vi "TABCheck.vi"(8 "Size":cluster{"X":dbl, "Y":dbl}, 9 "PtIn(Ideal/A)":cluster{"X":dbl, "Y":dbl}, 10 "Robot(B)":cluster{dbl, dbl}[][](array[cluster]), 11 "Ideal(A)":cluster{sgl, sgl}[][](array[cluster])) -> (3 "PtOut(Robot/B)":cluster{"OX":dbl, "OY":dbl})   [LabVIEW 2014]
panel:
  out "PointArray":cluster{"X":i32, "Y":i32}
  out "Array 2":cluster{i32, i32}[](array[cluster])
  out "Cluster":cluster{i32, i32}
  # "80,150"
  # "270,110"
  # "0,0"
  # "X,Y"
  # "107.5,160.8"
  # "0,1"
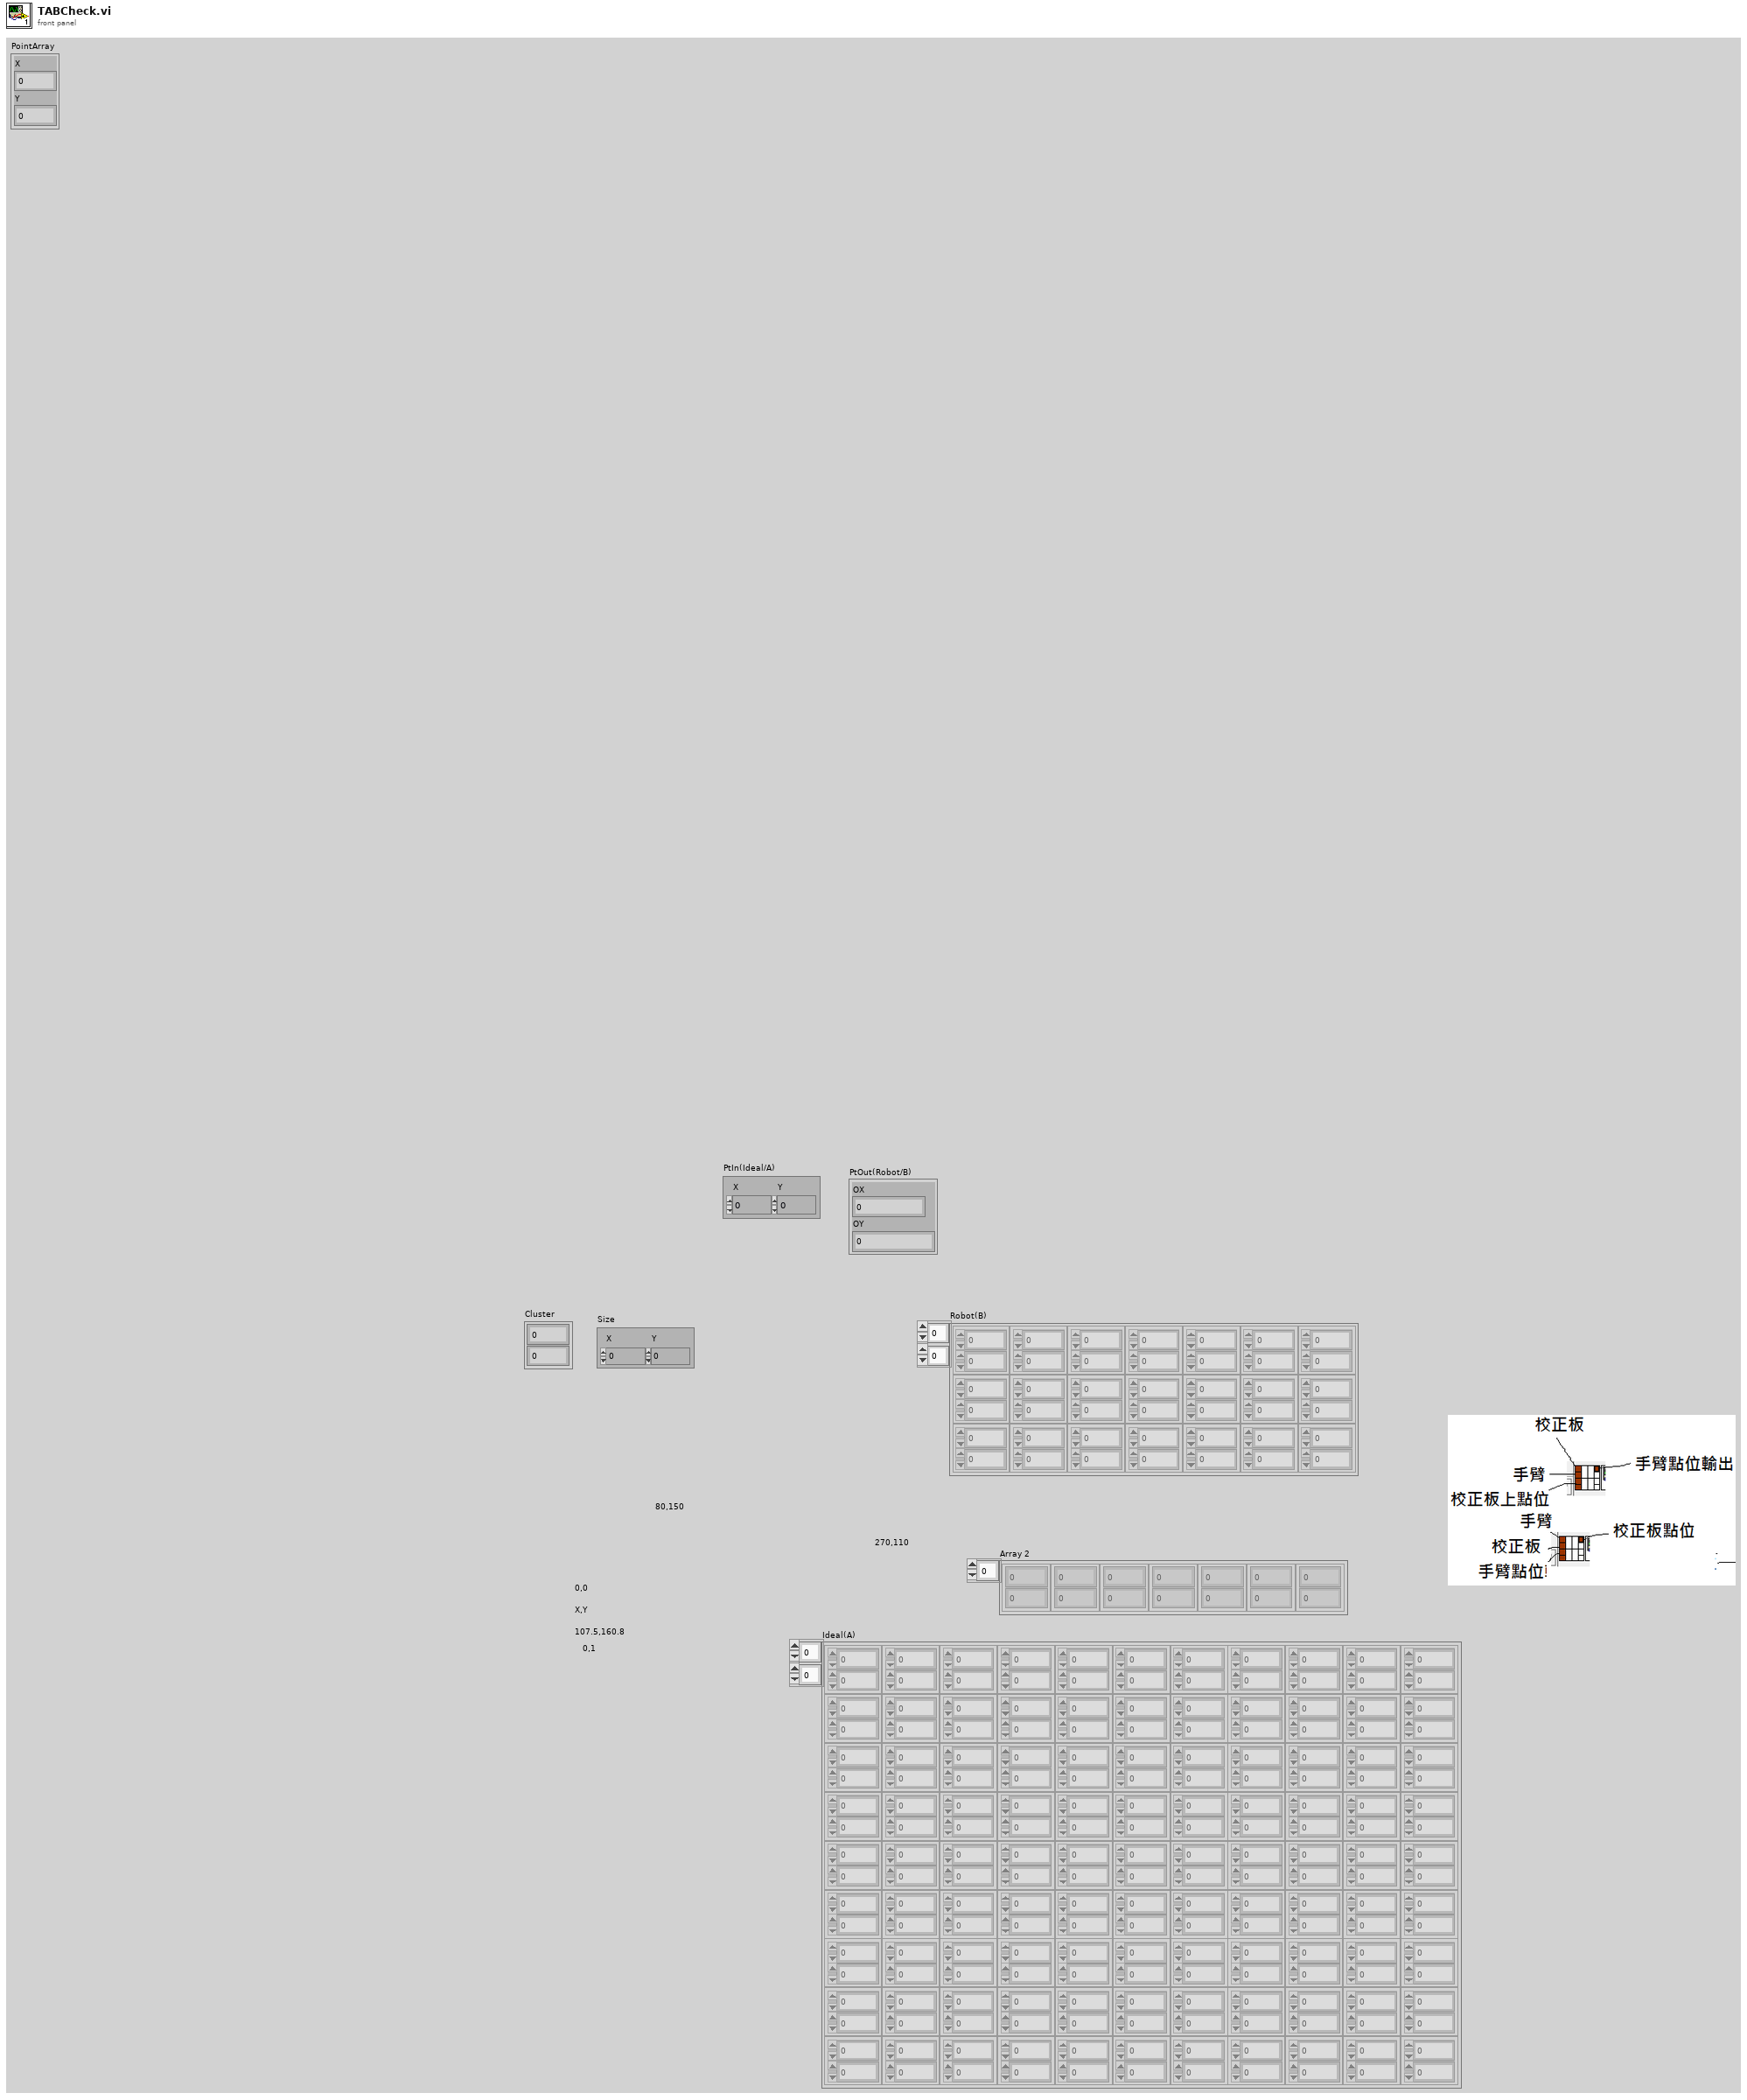
[diagram p1: front panel]
types:
  T1 = cluster{"[0]":sgl, "[1]":sgl, "[2]":sgl, "[3]":sgl}[]
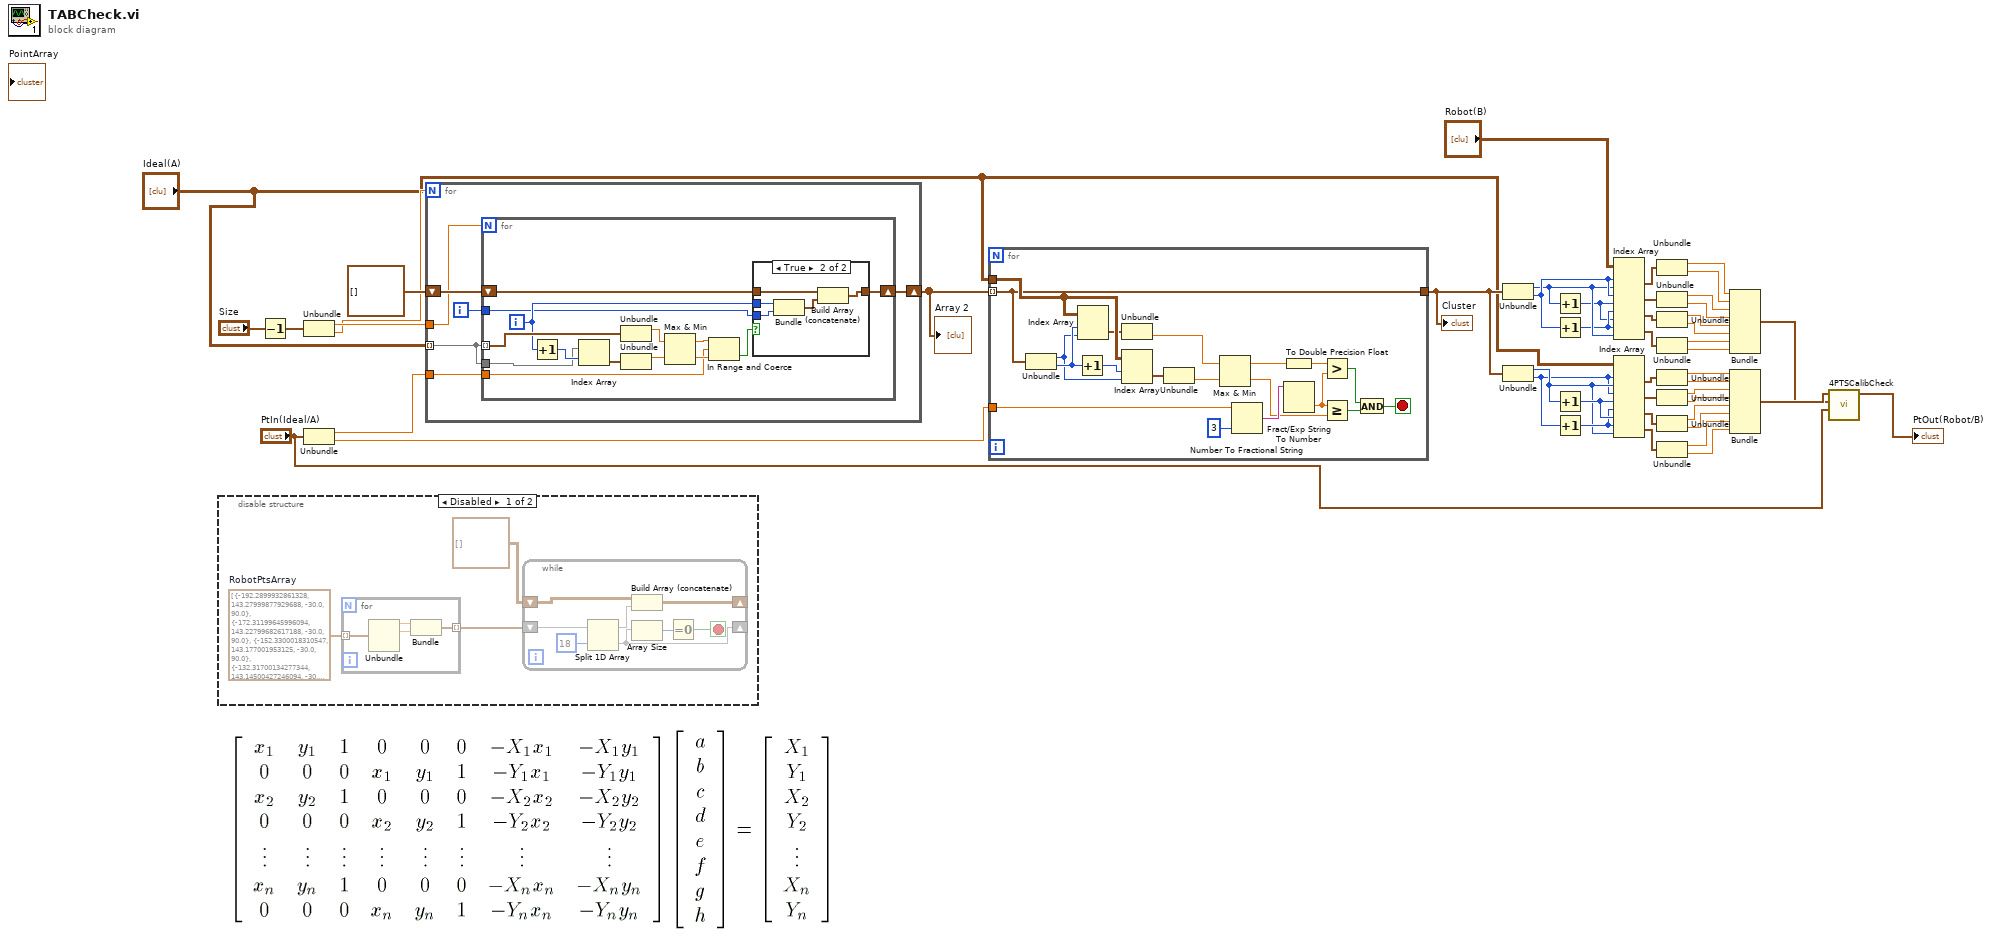
[diagram p0: block diagram]
diagram:
  n1 = disable-structure shown="Disabled" {
    frame Disabled {
      w49 = T1 [{"[0]"=-192.29, "[1]"=143.28, "[2]"=-30.0, "[3]"=90.0}, {"[0]"=-172.312, "[1]"=143.228, "[2]"=-30.0, "[3]"=90.0}, {"[0]"=-152.33, "[1]"=143.177, "[2]"=-30.0, "[3]"=90.0}, {"[0]"=-132.317, "[1]"=143.145, "[2]"=-30.0, "[3]"=90.0}, {"[0]"=-112.255, "[1]"=143.098, "[2]"=-30.0, "[3]"=90.0}, {"[0]"=-92.217, "[1]"=143.035, "[2]"=-30.0, "[3]"=90.0}, {"[0]"=-72.14, "[1]"=142.978, "[2]"=-30.0, "[3]"=90.0}, {"[0]"=-52.078, "[1]"=142.898, "[2]"=-30.0, "[3]"=90.0}, {"[0]"=-31.971, "[1]"=142.795, "[2]"=-30.0, "[3]"=90.0}, {"[0]"=-11.878, "[1]"=142.692, "[2]"=-30.0, "[3]"=90.0}, {"[0]"=8.277, "[1]"=142.568, "[2]"=-30.0, "[3]"=90.0}, {"[0]"=28.398, "[1]"=142.416, "[2]"=-30.0, "[3]"=90.0}, {"[0]"=48.523, "[1]"=142.253, "[2]"=-30.0, "[3]"=90.0}, {"[0]"=68.659, "[1]"=142.079, "[2]"=-30.0, "[3]"=90.0}, {"[0]"=88.714, "[1]"=141.902, "[2]"=-30.0, "[3]"=90.0}, {"[0]"=108.801, "[1]"=141.736, "[2]"=-30.0, "[3]"=90.0}, {"[0]"=128.813, "[1]"=141.58, "[2]"=-30.0, "[3]"=90.0}, {"[0]"=148.873, "[1]"=141.455, "[2]"=-30.0, "[3]"=90.0}, {"[0]"=-192.292, "[1]"=163.166, "[2]"=-30.0, "[3]"=90.0}, {"[0]"=-172.251, "[1]"=163.142, "[2]"=-30.0, "[3]"=90.0}, {"[0]"=-152.315, "[1]"=163.083, "[2]"=-30.0, "[3]"=90.0}, {"[0]"=-132.271, "[1]"=163.04, "[2]"=-30.0, "[3]"=90.0}, {"[0]"=-112.2, "[1]"=162.982, "[2]"=-30.0, "[3]"=90.0}, {"[0]"=-92.147, "[1]"=162.933, "[2]"=-30.0, "[3]"=90.0}, {"[0]"=-72.085, "[1]"=162.842, "[2]"=-30.0, "[3]"=90.0}, {"[0]"=-52.039, "[1]"=162.771, "[2]"=-30.0, "[3]"=90.0}, {"[0]"=-31.931, "[1]"=162.689, "[2]"=-30.0, "[3]"=90.0}, {"[0]"=-11.829, "[1]"=162.589, "[2]"=-30.0, "[3]"=90.0}, {"[0]"=8.306, "[1]"=162.465, "[2]"=-30.0, "[3]"=90.0}, {"[0]"=28.403, "[1]"=162.316, "[2]"=-30.0, "[3]"=90.0}, {"[0]"=48.518, "[1]"=162.165, "[2]"=-30.0, "[3]"=90.0}, {"[0]"=68.639, "[1]"=162.001, "[2]"=-30.0, "[3]"=90.0}, {"[0]"=88.711, "[1]"=161.847, "[2]"=-30.0, "[3]"=90.0}, {"[0]"=108.808, "[1]"=161.693, "[2]"=-30.0, "[3]"=90.0}, {"[0]"=128.797, "[1]"=161.532, "[2]"=-30.0, "[3]"=90.0}, {"[0]"=148.812, "[1]"=161.411, "[2]"=-30.0, "[3]"=90.0}, {"[0]"=-192.201, "[1]"=183.166, "[2]"=-30.0, "[3]"=90.0}, {"[0]"=-172.2, "[1]"=183.08, "[2]"=-30.0, "[3]"=90.0}, {"[0]"=-152.214, "[1]"=183.041, "[2]"=-30.0, "[3]"=90.0}, {"[0]"=-132.197, "[1]"=182.996, "[2]"=-30.0, "[3]"=90.0}, {"[0]"=-112.1, "[1]"=182.941, "[2]"=-30.0, "[3]"=90.0}, {"[0]"=-92.071, "[1]"=182.879, "[2]"=-30.0, "[3]"=90.0}, {"[0]"=-71.982, "[1]"=182.794, "[2]"=-30.0, "[3]"=90.0}, {"[0]"=-51.944, "[1]"=182.709, "[2]"=-30.0, "[3]"=90.0}, {"[0]"=-31.857, "[1]"=182.624, "[2]"=-30.0, "[3]"=90.0}, {"[0]"=-11.772, "[1]"=182.522, "[2]"=-30.0, "[3]"=90.0}, {"[0]"=8.361, "[1]"=182.426, "[2]"=-30.0, "[3]"=90.0}, {"[0]"=28.464, "[1]"=182.29, "[2]"=-30.0, "[3]"=90.0}, {"[0]"=48.542, "[1]"=182.127, "[2]"=-30.0, "[3]"=90.0}, {"[0]"=68.669, "[1]"=181.977, "[2]"=-30.0, "[3]"=90.0}, {"[0]"=88.728, "[1]"=181.825, "[2]"=-30.0, "[3]"=90.0}, {"[0]"=108.824, "[1]"=181.664, "[2]"=-30.0, "[3]"=90.0}, {"[0]"=128.779, "[1]"=181.533, "[2]"=-30.0, "[3]"=90.0}, {"[0]"=148.817, "[1]"=181.423, "[2]"=-30.0, "[3]"=90.0}, {"[0]"=-192.153, "[1]"=203.103, "[2]"=-30.0, "[3]"=90.0}, {"[0]"=-172.128, "[1]"=203.051, "[2]"=-30.0, "[3]"=90.0}, {"[0]"=-152.128, "[1]"=203.019, "[2]"=-30.0, "[3]"=90.0}, {"[0]"=-132.124, "[1]"=202.923, "[2]"=-30.0, "[3]"=90.0}, {"[0]"=-112.011, "[1]"=202.898, "[2]"=-30.0, "[3]"=90.0}, {"[0]"=-91.994, "[1]"=202.829, "[2]"=-30.0, "[3]"=90.0}, {"[0]"=-71.908, "[1]"=202.761, "[2]"=-30.0, "[3]"=90.0}, {"[0]"=-51.86, "[1]"=202.669, "[2]"=-30.0, "[3]"=90.0}, {"[0]"=-31.785, "[1]"=202.589, "[2]"=-30.0, "[3]"=90.0}, {"[0]"=-11.679, "[1]"=202.488, "[2]"=-30.0, "[3]"=90.0}, {"[0]"=8.407, "[1]"=202.38, "[2]"=-30.0, "[3]"=90.0}, {"[0]"=28.501, "[1]"=202.252, "[2]"=-30.0, "[3]"=90.0}, {"[0]"=48.585, "[1]"=202.111, "[2]"=-30.0, "[3]"=90.0}, {"[0]"=68.695, "[1]"=201.96, "[2]"=-30.0, "[3]"=90.0}, {"[0]"=88.739, "[1]"=201.807, "[2]"=-30.0, "[3]"=90.0}, {"[0]"=108.837, "[1]"=201.678, "[2]"=-30.0, "[3]"=90.0}, {"[0]"=128.774, "[1]"=201.553, "[2]"=-30.0, "[3]"=90.0}, {"[0]"=148.765, "[1]"=201.458, "[2]"=-30.0, "[3]"=90.0}, {"[0]"=-192.092, "[1]"=223.039, "[2]"=-30.0, "[3]"=90.0}, {"[0]"=-172.061, "[1]"=223.008, "[2]"=-30.0, "[3]"=90.0}, {"[0]"=-152.068, "[1]"=222.956, "[2]"=-30.0, "[3]"=90.0}, {"[0]"=-132.053, "[1]"=222.884, "[2]"=-30.0, "[3]"=90.0}, {"[0]"=-111.943, "[1]"=222.844, "[2]"=-30.0, "[3]"=90.0}, {"[0]"=-91.934, "[1]"=222.779, "[2]"=-30.0, "[3]"=90.0}, {"[0]"=-71.838, "[1]"=222.729, "[2]"=-30.0, "[3]"=90.0}, {"[0]"=-51.82, "[1]"=222.635, "[2]"=-30.0, "[3]"=90.0}, {"[0]"=-31.71, "[1]"=222.553, "[2]"=-30.0, "[3]"=90.0}, {"[0]"=-11.651, "[1]"=222.445, "[2]"=-30.0, "[3]"=90.0}, {"[0]"=8.465, "[1]"=222.341, "[2]"=-30.0, "[3]"=90.0}, {"[0]"=28.524, "[1]"=222.238, "[2]"=-30.0, "[3]"=90.0}, {"[0]"=48.613, "[1]"=222.096, "[2]"=-30.0, "[3]"=90.0}, {"[0]"=68.708, "[1]"=221.951, "[2]"=-30.0, "[3]"=90.0}, {"[0]"=88.759, "[1]"=221.807, "[2]"=-30.0, "[3]"=90.0}, {"[0]"=108.864, "[1]"=221.681, "[2]"=-30.0, "[3]"=90.0}, {"[0]"=128.728, "[1]"=221.571, "[2]"=-30.0, "[3]"=90.0}, {"[0]"=148.809, "[1]"=221.45, "[2]"=-30.0, "[3]"=90.0}, {"[0]"=-192.03, "[1]"=243.008, "[2]"=-30.0, "[3]"=90.0}, {"[0]"=-171.988, "[1]"=242.954, "[2]"=-30.0, "[3]"=90.0}, {"[0]"=-151.979, "[1]"=242.887, "[2]"=-30.0, "[3]"=90.0}, {"[0]"=-131.972, "[1]"=242.819, "[2]"=-30.0, "[3]"=90.0}, {"[0]"=-111.852, "[1]"=242.82, "[2]"=-30.0, "[3]"=90.0}, {"[0]"=-91.857, "[1]"=242.72, "[2]"=-30.0, "[3]"=90.0}, {"[0]"=-71.764, "[1]"=242.658, "[2]"=-30.0, "[3]"=90.0}, {"[0]"=-51.72, "[1]"=242.586, "[2]"=-30.0, "[3]"=90.0}, {"[0]"=-31.666, "[1]"=242.488, "[2]"=-30.0, "[3]"=90.0}, {"[0]"=-11.566, "[1]"=242.391, "[2]"=-30.0, "[3]"=90.0}, {"[0]"=8.484, "[1]"=242.29, "[2]"=-30.0, "[3]"=90.0}, {"[0]"=28.563, "[1]"=242.187, "[2]"=-30.0, "[3]"=90.0}, {"[0]"=48.663, "[1]"=242.057, "[2]"=-30.0, "[3]"=90.0}, {"[0]"=68.733, "[1]"=241.919, "[2]"=-30.0, "[3]"=90.0}, {"[0]"=88.775, "[1]"=241.787, "[2]"=-30.0, "[3]"=90.0}, {"[0]"=108.887, "[1]"=241.655, "[2]"=-30.0, "[3]"=90.0}, {"[0]"=128.678, "[1]"=241.573, "[2]"=-30.0, "[3]"=90.0}, {"[0]"=148.831, "[1]"=241.438, "[2]"=-30.0, "[3]"=90.0}, {"[0]"=-191.939, "[1]"=262.924, "[2]"=-30.0, "[3]"=90.0}, {"[0]"=-171.916, "[1]"=262.871, "[2]"=-30.0, "[3]"=90.0}, {"[0]"=-151.905, "[1]"=262.815, "[2]"=-30.0, "[3]"=90.0}, {"[0]"=-131.884, "[1]"=262.756, "[2]"=-30.0, "[3]"=90.0}, {"[0]"=-111.796, "[1]"=262.723, "[2]"=-30.0, "[3]"=90.0}, {"[0]"=-91.754, "[1]"=262.652, "[2]"=-30.0, "[3]"=90.0}, {"[0]"=-71.709, "[1]"=262.575, "[2]"=-30.0, "[3]"=90.0}, {"[0]"=-51.66, "[1]"=262.5, "[2]"=-30.0, "[3]"=90.0}, {"[0]"=-31.578, "[1]"=262.413, "[2]"=-30.0, "[3]"=90.0}, {"[0]"=-11.549, "[1]"=262.315, "[2]"=-30.0, "[3]"=90.0}, {"[0]"=8.537, "[1]"=262.228, "[2]"=-30.0, "[3]"=90.0}, {"[0]"=28.626, "[1]"=262.112, "[2]"=-30.0, "[3]"=90.0}, {"[0]"=48.685, "[1]"=261.99, "[2]"=-30.0, "[3]"=90.0}, {"[0]"=68.763, "[1]"=261.856, "[2]"=-30.0, "[3]"=90.0}, {"[0]"=88.802, "[1]"=261.731, "[2]"=-30.0, "[3]"=90.0}, {"[0]"=108.888, "[1]"=261.605, "[2]"=-30.0, "[3]"=90.0}, {"[0]"=128.724, "[1]"=261.511, "[2]"=-30.0, "[3]"=90.0}, {"[0]"=148.849, "[1]"=261.385, "[2]"=-30.0, "[3]"=90.0}, {"[0]"=-191.873, "[1]"=282.841, "[2]"=-30.0, "[3]"=90.0}, {"[0]"=-171.792, "[1]"=282.809, "[2]"=-30.0, "[3]"=90.0}, {"[0]"=-151.851, "[1]"=282.731, "[2]"=-30.0, "[3]"=90.0}, {"[0]"=-131.76, "[1]"=282.688, "[2]"=-30.0, "[3]"=90.0}, {"[0]"=-111.698, "[1]"=282.646, "[2]"=-30.0, "[3]"=90.0}, {"[0]"=-91.689, "[1]"=282.566, "[2]"=-30.0, "[3]"=90.0}, {"[0]"=-71.599, "[1]"=282.504, "[2]"=-30.0, "[3]"=90.0}, {"[0]"=-51.575, "[1]"=282.418, "[2]"=-30.0, "[3]"=90.0}, {"[0]"=-31.538, "[1]"=282.334, "[2]"=-30.0, "[3]"=90.0}, {"[0]"=-11.474, "[1]"=282.248, "[2]"=-30.0, "[3]"=90.0}, {"[0]"=8.619, "[1]"=282.156, "[2]"=-30.0, "[3]"=90.0}, {"[0]"=28.696, "[1]"=282.05, "[2]"=-30.0, "[3]"=90.0}, {"[0]"=48.729, "[1]"=281.927, "[2]"=-30.0, "[3]"=90.0}, {"[0]"=68.834, "[1]"=281.809, "[2]"=-30.0, "[3]"=90.0}, {"[0]"=88.829, "[1]"=281.684, "[2]"=-30.0, "[3]"=90.0}, {"[0]"=108.776, "[1]"=281.592, "[2]"=-30.0, "[3]"=90.0}, {"[0]"=128.746, "[1]"=281.476, "[2]"=-30.0, "[3]"=90.0}, {"[0]"=148.9, "[1]"=281.337, "[2]"=-30.0, "[3]"=90.0}]  # RobotPtsArray
      n2 = for {
        tunnel: w49 -> [w54] mode=indexing
        tunnel: [w51] -> w48 mode=indexing
        n3 = Unbundle(w54) -> ("[0]"=w53:sgl, "[1]"=w52:sgl)  [unwired: 2 out]
        n4 = Bundle("[0]"=w53, "[1]"=w52) -> (w51:cluster{"[0]":sgl, "[1]":sgl})  [unwired: 1 in]
      }
      n5 = while {
        shift-right: [w60] -> _
        shift-left: w48 -> [w62]
        shift-right: [w56] -> _
        shift-left: cluster{"[0]":sgl, "[1]":sgl}[][] [] -> [w55]
        stop <- w58 stop-if-true
        n6 = Split 1D Array(array=w62, index=18) -> (first subarray=w57:cluster{"[0]":sgl, "[1]":sgl}[], second subarray=w60:cluster{"[0]":sgl, "[1]":sgl}[])
        n7 = Build Array (concatenate)(w55, w57) -> (w56:cluster{"[0]":sgl, "[1]":sgl}[][])
        n8 = Array Size(array=w60) -> (size(s)=w59:i32)
        n9 = Equal To 0?(x=w59) -> (x = 0?=w58:bool)
      }
    }
    frame Enabled {
    }
  }
  n10 = Decrement(x="Size") -> (x-1=w43:cluster{"X":dbl, "Y":dbl})
  n11 = Unbundle(w43) -> ("X"=w42:dbl, "Y"=w41:dbl)
  n12 = Unbundle("PtIn(Ideal/A)") -> ("X"=w47:dbl, "Y"=w44:dbl)
  n13 = for {
    N: w41 -> [_]
    tunnel: w47 -> [w68]
    tunnel: "Ideal(A)" -> [w67] mode=indexing
    shift-right: [w64] -> w45
    shift-left: cluster{i32, i32}[] [] -> [w65]
    tunnel: w42 -> [w63]
    i -> [w66]
    n14 = for {
      N: w63 -> [_]
      tunnel: w67 -> [w82] mode=indexing
      tunnel: w67 -> [w69]
      tunnel: w68 -> [w75]
      tunnel: w66 -> [w73]
      shift-right: [w72] -> w64
      shift-left: w65 -> [w71]
      i -> [w74]
      n15 = Increment(x=w74) -> (x+1=w81:i32)
      n16 = Index Array(array=w69, index=w81) -> (element=w80:cluster{sgl, sgl})
      n17 = Unbundle(w82) -> (w79:sgl)  [unwired: 1 out]
      n18 = Unbundle(w80) -> (w78:sgl)  [unwired: 1 out]
      n19 = Max & Min(x=w79, y=w78) -> (max(x,y)=w77:sgl, min(x,y)=w76:sgl)
      n20 = In Range and Coerce(upper limit=w77, x=w75, lower limit=w76) -> (In Range?=w70:bool)  [unwired: 1 out]
      n21 = case shown="True" w70 {
        tunnel: w74 -> [_ w88]
        tunnel: w73 -> [_ w87]
        tunnel: [w83 w85] -> w72
        tunnel: w71 -> [w83 w84]
        frame False {
        }
        frame True {
          n22 = Bundle(w88, w87) -> (w86:cluster{i32, i32})  [unwired: 1 in]
          n23 = Build Array (concatenate)(w84, w86) -> (w85:cluster{i32, i32}[])
        }
      }
    }
  }
  "Array 2" <- w45
  n24 = for {
    tunnel: "Ideal(A)" -> [w107]
    tunnel: w45 -> [w102] mode=indexing
    tunnel: w44 -> [w94]
    tunnel: [w102] -> w19
    stop <- w95 stop-if-true
    n25 = Unbundle(w102) -> (w99:i32, w100:i32)
    n26 = Increment(x=w100) -> (x+1=w101:i32)
    n27 = Index Array(array=w107, index (row)=w100, index (col)=w99) -> (element=w106:cluster{sgl, sgl})
    n28 = Unbundle(w106) -> (w104:sgl)  [unwired: 1 out]
    n29 = Index Array(array=w107, index (row)=w101, index (col)=w99) -> (element=w105:cluster{sgl, sgl})
    n30 = Unbundle(w105) -> (w103:sgl)  [unwired: 1 out]
    n31 = Max & Min(x=w104, y=w103) -> (max(x,y)=w98:sgl, min(x,y)=w90:sgl)
    n32 = Number To Fractional String(number=w94, precision (6)=i16 3) -> (F-format string=w92:string)  [unwired: 2 in]
    n33 = To Double Precision Float(number=w98) -> (double precision float=w97:dbl)
    n34 = Fract/Exp String To Number(string=w92) -> (number=w91:dbl)  [unwired: 3 in, 1 out]
    n35 = Greater?(x=w97, y=w91) -> (0:w96:bool)
    n36 = Greater Or Equal?(x=w91, y=w90) -> (x >= y?=w89:bool)
    n37 = And(x=w96, y=w89) -> (x .and. y?=w95:bool)
  }
  "Cluster" <- w19
  n38 = Unbundle(w19) -> (w22:i32, w23:i32)
  n39 = Unbundle(w19) -> (w25:i32, w24:i32)
  n40 = Increment(x=w22) -> (x+1=w20:i32)
  n41 = Increment(x=w23) -> (x+1=w21:i32)
  n42 = Increment(x=w25) -> (x+1=w39:i32)
  n43 = Increment(x=w24) -> (x+1=w38:i32)
  n44 = Index Array(array="Robot(B)", index (row) #1=w23, index (col) #1=w22, index (row) #2=w23, index (col) #2=w20, index (row) #3=w21, index (col) #3=w20, index (row) #4=w21, index (col) #4=w22) -> (element #1=w11:cluster{dbl, dbl}, element #2=w10:cluster{dbl, dbl}, element #3=w9:cluster{dbl, dbl}, element #4=w8:cluster{dbl, dbl})
  n45 = Index Array(array="Ideal(A)", index (row) #1=w24, index (col) #1=w25, index (row) #2=w24, index (col) #2=w39, index (row) #3=w38, index (col) #3=w39, index (row) #4=w38, index (col) #4=w25) -> (element #1=w37:cluster{sgl, sgl}, element #2=w36:cluster{sgl, sgl}, element #3=w35:cluster{sgl, sgl}, element #4=w34:cluster{sgl, sgl})
  n46 = Unbundle(w11) -> (w12:dbl, w13:dbl)
  n47 = Unbundle(w10) -> (w14:dbl, w15:dbl)
  n48 = Unbundle(w9) -> (w16:dbl, w17:dbl)
  n49 = Unbundle(w8) -> (w18:dbl, w7:dbl)
  n50 = Unbundle(w37) -> (w33:sgl, w32:sgl)
  n51 = Unbundle(w36) -> (w31:sgl, w30:sgl)
  n52 = Unbundle(w35) -> (w29:sgl, w28:sgl)
  n53 = Unbundle(w34) -> (w27:sgl, w26:sgl)
  n54 = Bundle(w12, w13, w14, w15, w16, w17, w18, w7) -> (w1:cluster{dbl, dbl, dbl, dbl, dbl, dbl, dbl, dbl})  [unwired: 1 in]
  n55 = Bundle(w33, w32, w31, w30, w29, w28, w27, w26) -> (w2:cluster{sgl, sgl, sgl, sgl, sgl, sgl, sgl, sgl})  [unwired: 1 in]
  n56 = call "4PTSCalibCheck.vi"("IdealPointIn(A)"="PtIn(Ideal/A)", "InputRobot(B)"=w1, "InputIdeal(A)"=w2) -> ("RobotOut(B )"=→"PtOut(Robot/B)":cluster{"RX":dbl, "RY":dbl})  [unwired: 8 in]
